vi "Set guard interval.vi"(8 "error in (no error)":errorcluster, 10 "Guard Interval":T1=enum."SHORT" caption="GI", 11 "niDTS WLAN Dut in":refnum<class "niDTS WLAN Dut.lvclass">) -> (0 "error out":errorcluster, 3 "niDTS WLAN Dut out":refnum<class "niDTS WLAN Dut.lvclass">)   [LabVIEW 2015, in "niDTS WLAN.lvlib" / "niDTS WLAN Dut.lvclass"]
uses:
  niDTS WLAN Dut.lvclass
  Includes/niDTS WLAN INC GI.ctl
  niDTS WLAN Dut.lvclass/niDTS WLAN Dut.ctl
  niDTS WLAN.lvlib
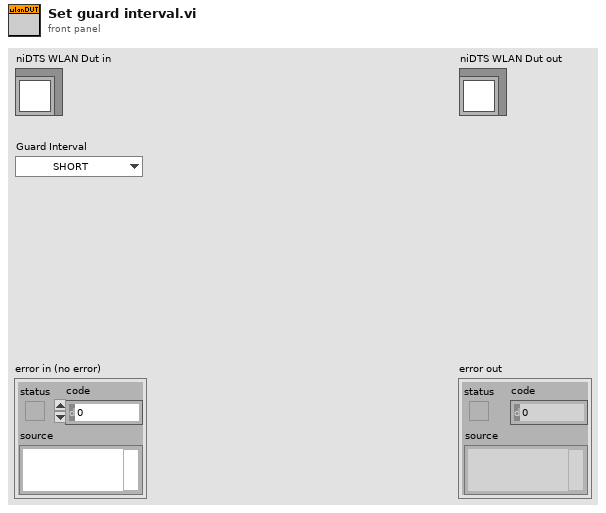
[diagram p1: front panel]
types:
  T1 = typedef "niDTS WLAN.lvlib/niDTS WLAN INC GI.ctl" = enum16{"LONG", "SHORT"}
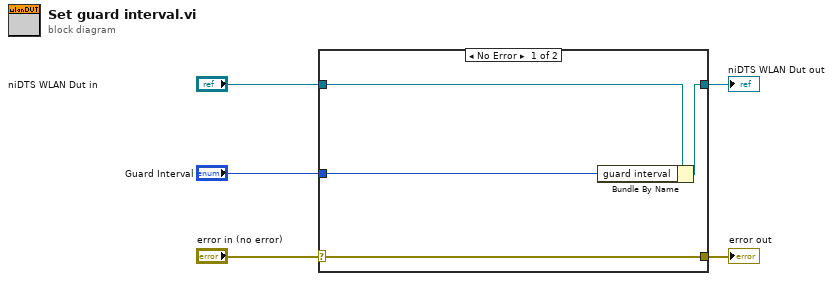
[diagram p0: block diagram]
diagram:
  n1 = case shown="No Error" "error in (no error)" {
    selector: "error in (no error)" -> [w9 w10]
    tunnel: [w9 w10] -> w4
    tunnel: [w7 w11] -> w2
    tunnel: "niDTS WLAN Dut in" -> [w8 w11]
    tunnel: "Guard Interval" -> [w6 _]
    frame No Error {
      n2 = Bundle By Name(cluster=w8, "guard interval"=w6) -> (w7:refnum<class "niDTS WLAN Dut.lvclass">)
    }
    frame Error {
    }
  }
  "error out" <- w4
  "niDTS WLAN Dut out" <- w2
